vi "Odometry Set.vi"() -> ()   [LabVIEW 2019]
uses:
  <vilib>/Rock Robotics/WPI/ThirdParty/WPILib Extensions/Geometry/Typedef/Pose2d.ctl
  <vilib>/Rock Robotics/WPI/ThirdParty/WPILib Extensions/Geometry/Typedef/Translation2d.ctl
  <vilib>/Rock Robotics/WPI/ThirdParty/WPILib Extensions/Geometry/Typedef/Rotation2d.ctl
panel:
  in  "Pose2d":T1
  in  "Set?":bool
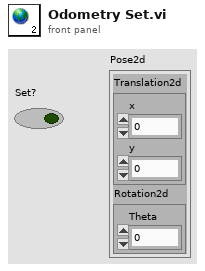
[diagram p1: front panel]
types:
  T1 = typedef "Pose2d.ctl" = cluster{"Translation2d":T2, "Rotation2d":T3}
  T2 = typedef "Translation2d.ctl" = cluster{"x":dbl, "y":dbl}
  T3 = typedef "Rotation2d.ctl" = cluster{"Theta":dbl}
diagram:
